vi "AuMT8852B Max Input Power Configuration.vi"(5 "Settings":T1={"Low frequency selection"=enum."Use low frequency", "Medium frequency selection"=enum."Use medium frequency", "High frequency selection"=enum."Use high frequency", "Low TX frequency"=2480.0, "Low RX frequency"=2402.0, "Medium TX frequency"=2402.0, "Medium RX frequency"=2441.0, "High TX frequency"=2402.0, "High RX frequency"=2480.0, "Number of packets"=7408, "Test TX power"=-20.0, "BER limit"=0.1, "FER limit"=100.0, "Packet count"=enum."TX"} {"FER limit" format="%.2f"; "BER limit" format="%.2f"; "Test TX power" format="%.1f"}, 7 "Set/Get (Set)":enum16{"Set", "Get"}(ring), 8 "error in (no error)":errorcluster, 10 "Script (3)":i32=3, 11 "VISA session":refnum<visa-resource-name>) -> (0 "error out":errorcluster, 2 "error code":i32, 3 "VISA session out":refnum<visa-resource-name>, 4 "Settings out":T1={"Low frequency selection"=enum."Use low frequency", "Medium frequency selection"=enum."Use medium frequency", "High frequency selection"=enum."Use high frequency", "Low TX frequency"=0.0, "Low RX frequency"=0.0, "Medium TX frequency"=0.0, "Medium RX frequency"=0.0, "High TX frequency"=0.0, "High RX frequency"=0.0, "Number of packets"=0, "Test TX power"=0.0, "BER limit"=0.0, "FER limit"=0.0, "Packet count"=enum."TX"} {"FER limit" format="%.2f"; "BER limit" format="%.2f"; "Test TX power" format="%.1f"})   [LabVIEW 2017]
doc: "Anritsu MT8852B Bluetooth Tester\n\nConfigures the instrument for the Maximum Input Power Sensitivity test.\n\nINPUTS\nSet/Get - whether the values are being sent to or retrieved from the instrument.\nScript - which of the stored scripts (1-10) will be queried or configured. Scripts 1 and 2 are read-only.\nSettings - parameters of the test to be written.\n\nOUTPUTS\nSettings out - current parameters of the test."
uses:
  <instrlib>/aumt8852B/General/Utilities/MT8850 Test Parameters.ctl
  <instrlib>/aumt8852B/General/Utilities/MT8850 Frequency Units.ctl
panel:
  in  "Case Constant\n(See Context Help)":bool
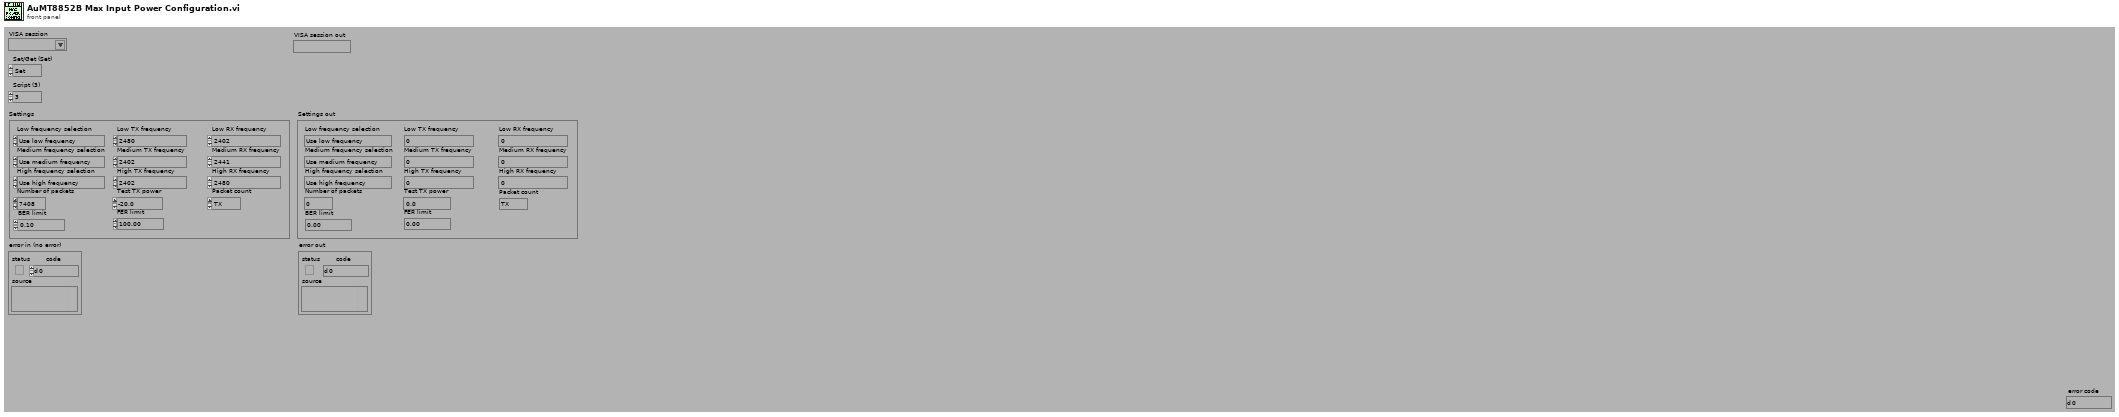
[diagram p1: front panel]
types:
  T1 = cluster{"Low frequency selection":enum16{"Don't use low frequency", "Use low frequency"}, "Medium frequency selection":enum16{"Don't use medium frequency", "Use medium frequency"}, "High frequency selection":enum16{"Don't use high frequency", "Use high frequency"}, "Low TX frequency":dbl, "Low RX frequency":dbl, "Medium TX frequency":dbl, "Medium RX frequency":dbl, "High TX frequency":dbl, "High RX frequency":dbl, "Number of packets":i32, "Test TX power":dbl, "BER limit":dbl, "FER limit":dbl, "Packet count":enum16{"TX", "RX"}}
  T2 = typedef "MT8850 Test Parameters.ctl" = enum16{"Use low frequency", "Use medium frequency", "Use high frequency", "Low TX frequency", "Low RX frquency", "Medium TX frequency", "Medium RX frequency", "High TX frequency", "High RX frequency", "Number of packets", "Average high limit", "Average low limit", "Peak power limit", "Max power step limit", "Min power step limit", "f1 average minimum", "f1 average maximum", "f2 maximum", "f1/f2 average maximum", "Hop selection", "Use DH1 packets", "Use DH3 packets", "Use DH5 packets", "1 slot packet drift limit", "3 slot packet drift limit", "5 slot packet drift limit", "Drift rate limit", "TX power level", "Frequency offset", "Symbol timing", "Modulation index", "BER limit", "FER limit", "Use averaging high limit", "Use averaging low limit", "Use peak power limit", "Packet type", "Test control", "Use max power step limit", "Use min power step limit", "Number of cycles", "Use f1 average maximum", "Use f1 average minimum", "Use f2 maximum", "Use f1/f2 average maximum", "Hop mode", "Maximum negative limit", "Maximum positive limit", "Use maximum negative limit", "Use maximum positive limit", "Use 1 slot packet drift limit", "Use 3 slot packet drift limit", "Use 5 slot packet drift limit", "Use drift rate limit", "Use BER limit", "Use FER limit", "Use dirty parameter table", "Use null packet drift limit", "Null packet drift limit", "Minimum power", "Power delay", "Packet count", "Payload toggle", "Output power level", "2DHX packet type", "3DHX packet type", "Number of blocks", "TX and RX low frequency", "TX and RX medium frequency", "TX and RX high frequency", "TX frequency", "RX frequency", "Threshold bit count", "Total test bit count", "Number of bits", "PDPSK to PGFSK lower limit", "PDPSK to PGFSK upper limit", "Initial frequency error upper limit", "Initial frequency error lower limit", "Frequency error upper limit", "Frequency error lower limit", "Block frequency error upper limit", "Block frequency error lower limit", "2Mbs RMS DEVM limit", "3Mbs RMS DEVM limit", "2Mbs Peak DEVM limit", "3Mbs Peak DEVM limit", "2Mbs 99% packets DEVM limit", "3Mbs 99% packets DEVM limit", "Percentage of no error packets limit", "Threshold error limit", "Total test error limit"}
  T3 = typedef "MT8850 Frequency Units.ctl" = enum16{"Channel", "Hz", "kHz", "MHz", "GHz"}
  T4 = enum16{"Simulate", "Range check", "Cache", "Query instrument status"}
  T5 = enum16{"Output power", "Power control", "Modulation characteristics", "Initial carrier", "Carrier drift", "Single slot sensitivity", "Multiple slot sensitivity", "Maximum input power"}
  T6 = enum16{"Don't use high frequency", "Use high frequency"}
  T7 = enum16{"Don't use medium frequency", "Use medium frequency"}
  T8 = enum16{"Don't use low frequency", "Use low frequency"}
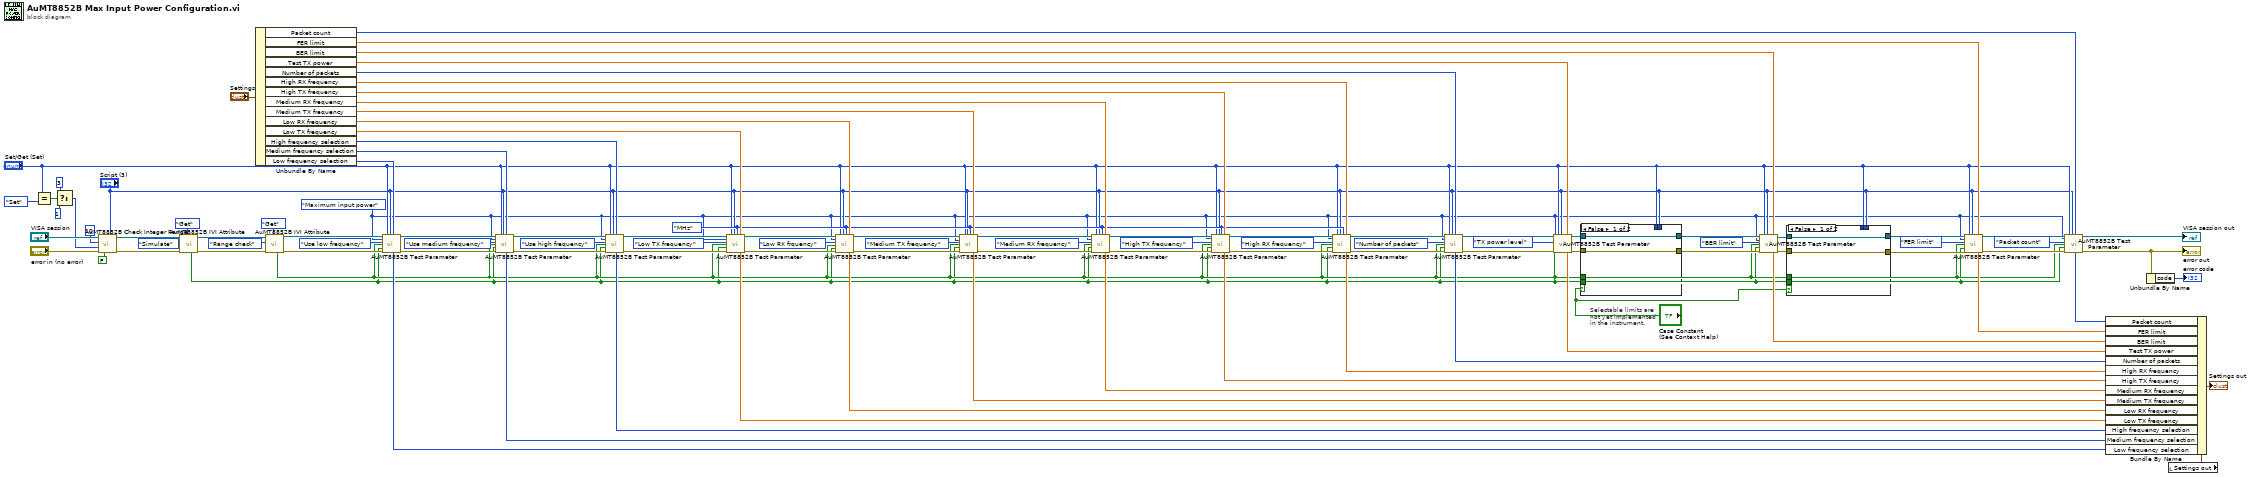
[diagram p0: block diagram]
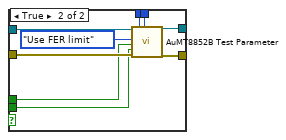
[diagram p2: hidden frame]
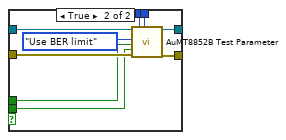
[diagram p3: hidden frame]
diagram:
  w13 = MT8850_Frequency_Units."MHz" ("Frequency units (MHz)")
  w2 = T5."Maximum input power" ("Test (Output Power)")
  # "Selectable limits are\nnot yet implemented\nin the instrument."
  n1 = Equal?(x="Set/Get (Set)", y=enum16{"Set", "Get"}."Set") -> (x = y?=w101:bool)
  n2 = Select(t=3, s=w101, f=1) -> (s? t:f=w97:i32)
  n3 = call <instrlib>:"AuMT8852B Check Integer Range.vi"("Value (0)"="Script (3)", "Check IVI flag first? (T)"=FALSE, "error in (no error)"="error in (no error)", "Lower limit (-1)"=w97, "Upper limit (1)"=10, "VISA session"="VISA session") -> ("error out"=w95:errorcluster, "VISA session out"=w96:refnum<visa-resource-name>)  [unwired: 4 in]
  n4 = call <instrlib>:"AuMT8852B IVI Attribute.vi"("Set/Get (Set)"=enum16{"Set", "Get"}."Get", "error in (no error)"=w95, "Flag (Simulate)"=T4."Simulate", "VISA session"=w96) -> ("error out"=w69:errorcluster, "VISA session out"=w70:refnum<visa-resource-name>, "Value out"=w8:bool)  [unwired: 5 in]
  n5 = Unbundle By Name("Settings") -> ("Packet count"=w1:enum16{"TX", "RX"}, "FER limit"=w37:dbl, "BER limit"=w38:dbl, "Test TX power"=w42:dbl, "Number of packets"=w43:i32, "High RX frequency"=w56:dbl, "High TX frequency"=w57:dbl, "Medium RX frequency"=w44:dbl, "Medium TX frequency"=w58:dbl, "Low RX frequency"=w59:dbl, "Low TX frequency"=w60:dbl, "High frequency selection"=w61:T6, "Medium frequency selection"=w62:T7, "Low frequency selection"=w63:T8)
  n6 = call <instrlib>:"AuMT8852B IVI Attribute.vi"("Set/Get (Set)"=enum16{"Set", "Get"}."Get", "error in (no error)"=w69, "Flag (Simulate)"=T4."Range check", "VISA session"=w70) -> ("error out"=w67:errorcluster, "VISA session out"=w68:refnum<visa-resource-name>, "Value out"=w9:bool)  [unwired: 5 in]
  n7 = call <instrlib>:"AuMT8852B Test Parameter.vi"("VISA session"=w68, "Test (Output power)"=w2, "Parameter (Use low frequency)"=MT8850_Test_Parameters."Use low frequency", "Range check? (F)"=w9, "Simulate? (F)"=w8, "error in (no error)"=w67, "Set/Get (Set)"="Set/Get (Set)", "Script (3)"="Script (3)", "Integer value (0)"=w63) -> ("Integer value out"=w48:i32, "VISA session out"=w20:refnum<visa-resource-name>, "error out"=w19:errorcluster)  [unwired: 7 in, 1 out]
  n8 = call <instrlib>:"AuMT8852B Test Parameter.vi"("VISA session"=w20, "Test (Output power)"=w2, "Parameter (Use low frequency)"=MT8850_Test_Parameters."Use medium frequency", "Range check? (F)"=w9, "Simulate? (F)"=w8, "error in (no error)"=w19, "Set/Get (Set)"="Set/Get (Set)", "Script (3)"="Script (3)", "Integer value (0)"=w62) -> ("Integer value out"=w49:i32, "VISA session out"=w18:refnum<visa-resource-name>, "error out"=w17:errorcluster)  [unwired: 7 in, 1 out]
  n9 = call <instrlib>:"AuMT8852B Test Parameter.vi"("VISA session"=w18, "Test (Output power)"=w2, "Parameter (Use low frequency)"=MT8850_Test_Parameters."Use high frequency", "Range check? (F)"=w9, "Simulate? (F)"=w8, "error in (no error)"=w17, "Set/Get (Set)"="Set/Get (Set)", "Script (3)"="Script (3)", "Integer value (0)"=w61) -> ("Integer value out"=w50:i32, "VISA session out"=w91:refnum<visa-resource-name>, "error out"=w90:errorcluster)  [unwired: 7 in, 1 out]
  n10 = call <instrlib>:"AuMT8852B Test Parameter.vi"("VISA session"=w91, "Test (Output power)"=w2, "Parameter (Use low frequency)"=MT8850_Test_Parameters."Low TX frequency", "Range check? (F)"=w9, "Simulate? (F)"=w8, "error in (no error)"=w90, "Set/Get (Set)"="Set/Get (Set)", "Script (3)"="Script (3)", "Integer value (0)"=w13, "Float value (0)"=w60) -> ("Float value out"=w51:dbl, "VISA session out"=w89:refnum<visa-resource-name>, "error out"=w88:errorcluster)  [unwired: 6 in, 1 out]
  n11 = call <instrlib>:"AuMT8852B Test Parameter.vi"("VISA session"=w89, "Test (Output power)"=w2, "Parameter (Use low frequency)"=MT8850_Test_Parameters."Low RX frquency", "Range check? (F)"=w9, "Simulate? (F)"=w8, "error in (no error)"=w88, "Set/Get (Set)"="Set/Get (Set)", "Script (3)"="Script (3)", "Integer value (0)"=w13, "Float value (0)"=w59) -> ("Float value out"=w52:dbl, "VISA session out"=w87:refnum<visa-resource-name>, "error out"=w86:errorcluster)  [unwired: 6 in, 1 out]
  n12 = call <instrlib>:"AuMT8852B Test Parameter.vi"("VISA session"=w87, "Test (Output power)"=w2, "Parameter (Use low frequency)"=MT8850_Test_Parameters."Medium TX frequency", "Range check? (F)"=w9, "Simulate? (F)"=w8, "error in (no error)"=w86, "Set/Get (Set)"="Set/Get (Set)", "Script (3)"="Script (3)", "Integer value (0)"=w13, "Float value (0)"=w58) -> ("Float value out"=w53:dbl, "VISA session out"=w85:refnum<visa-resource-name>, "error out"=w84:errorcluster)  [unwired: 6 in, 1 out]
  n13 = call <instrlib>:"AuMT8852B Test Parameter.vi"("VISA session"=w85, "Test (Output power)"=w2, "Parameter (Use low frequency)"=MT8850_Test_Parameters."Medium RX frequency", "Range check? (F)"=w9, "Simulate? (F)"=w8, "error in (no error)"=w84, "Set/Get (Set)"="Set/Get (Set)", "Script (3)"="Script (3)", "Integer value (0)"=w13, "Float value (0)"=w44) -> ("Float value out"=w46:dbl, "VISA session out"=w83:refnum<visa-resource-name>, "error out"=w82:errorcluster)  [unwired: 6 in, 1 out]
  n14 = call <instrlib>:"AuMT8852B Test Parameter.vi"("VISA session"=w83, "Test (Output power)"=w2, "Parameter (Use low frequency)"=MT8850_Test_Parameters."High TX frequency", "Range check? (F)"=w9, "Simulate? (F)"=w8, "error in (no error)"=w82, "Set/Get (Set)"="Set/Get (Set)", "Script (3)"="Script (3)", "Integer value (0)"=w13, "Float value (0)"=w57) -> ("Float value out"=w54:dbl, "VISA session out"=w81:refnum<visa-resource-name>, "error out"=w80:errorcluster)  [unwired: 6 in, 1 out]
  n15 = call <instrlib>:"AuMT8852B Test Parameter.vi"("VISA session"=w81, "Test (Output power)"=w2, "Parameter (Use low frequency)"=MT8850_Test_Parameters."High RX frequency", "Range check? (F)"=w9, "Simulate? (F)"=w8, "error in (no error)"=w80, "Set/Get (Set)"="Set/Get (Set)", "Script (3)"="Script (3)", "Integer value (0)"=w13, "Float value (0)"=w56) -> ("Float value out"=w55:dbl, "VISA session out"=w79:refnum<visa-resource-name>, "error out"=w78:errorcluster)  [unwired: 6 in, 1 out]
  n16 = call <instrlib>:"AuMT8852B Test Parameter.vi"("VISA session"=w79, "Test (Output power)"=w2, "Parameter (Use low frequency)"=MT8850_Test_Parameters."Number of packets", "Range check? (F)"=w9, "Simulate? (F)"=w8, "error in (no error)"=w78, "Set/Get (Set)"="Set/Get (Set)", "Script (3)"="Script (3)", "Integer value (0)"=w43) -> ("Integer value out"=w45:i32, "VISA session out"=w33:refnum<visa-resource-name>, "error out"=w32:errorcluster)  [unwired: 7 in, 1 out]
  n17 = call <instrlib>:"AuMT8852B Test Parameter.vi"("VISA session"=w33, "Test (Output power)"=w2, "Parameter (Use low frequency)"=MT8850_Test_Parameters."TX power level", "Range check? (F)"=w9, "Simulate? (F)"=w8, "error in (no error)"=w32, "Set/Get (Set)"="Set/Get (Set)", "Script (3)"="Script (3)", "Float value (0)"=w42) -> ("Float value out"=w36:dbl, "VISA session out"=w26:refnum<visa-resource-name>, "error out"=w23:errorcluster)  [unwired: 7 in, 1 out]
  n18 = case shown="False" "Case Constant\n(See Context Help)" {
    tunnel: w26 -> [w106 w114]
    tunnel: [w106 w113] -> w25
    tunnel: [w105 w112] -> w24
    tunnel: w23 -> [w105 w111]
    tunnel: w9 -> [_ w110]
    tunnel: w8 -> [_ w109]
    tunnel: "Set/Get (Set)" -> [_ w108]
    tunnel: "Script (3)" -> [_ w107]
    frame False {
    }
    frame True {
      n19 = call <instrlib>:"AuMT8852B Test Parameter.vi"("VISA session"=w114, "Parameter (Use low frequency)"=MT8850_Test_Parameters."Use BER limit", "Range check? (F)"=w110, "Simulate? (F)"=w109, "error in (no error)"=w111, "Set/Get (Set)"=w108, "Script (3)"=w107) -> ("VISA session out"=w113:refnum<visa-resource-name>, "error out"=w112:errorcluster)  [unwired: 9 in, 2 out]
    }
  }
  n20 = call <instrlib>:"AuMT8852B Test Parameter.vi"("VISA session"=w25, "Test (Output power)"=w2, "Parameter (Use low frequency)"=MT8850_Test_Parameters."BER limit", "Range check? (F)"=w9, "Simulate? (F)"=w8, "error in (no error)"=w24, "Set/Get (Set)"="Set/Get (Set)", "Script (3)"="Script (3)", "Float value (0)"=w38) -> ("Float value out"=w35:dbl, "VISA session out"=w30:refnum<visa-resource-name>, "error out"=w29:errorcluster)  [unwired: 7 in, 1 out]
  n21 = case shown="False" "Case Constant\n(See Context Help)" {
    tunnel: w30 -> [w116 w125]
    tunnel: w29 -> [w117 w124]
    tunnel: [w116 w123] -> w28
    tunnel: [w117 w122] -> w27
    tunnel: w9 -> [_ w121]
    tunnel: w8 -> [_ w120]
    tunnel: "Set/Get (Set)" -> [_ w119]
    tunnel: "Script (3)" -> [_ w118]
    frame False {
    }
    frame True {
      n22 = call <instrlib>:"AuMT8852B Test Parameter.vi"("VISA session"=w125, "Parameter (Use low frequency)"=MT8850_Test_Parameters."Use FER limit", "Range check? (F)"=w121, "Simulate? (F)"=w120, "error in (no error)"=w124, "Set/Get (Set)"=w119, "Script (3)"=w118) -> ("VISA session out"=w123:refnum<visa-resource-name>, "error out"=w122:errorcluster)  [unwired: 9 in, 2 out]
    }
  }
  n23 = call <instrlib>:"AuMT8852B Test Parameter.vi"("VISA session"=w28, "Test (Output power)"=w2, "Parameter (Use low frequency)"=MT8850_Test_Parameters."FER limit", "Range check? (F)"=w9, "Simulate? (F)"=w8, "error in (no error)"=w27, "Set/Get (Set)"="Set/Get (Set)", "Script (3)"="Script (3)", "Float value (0)"=w37) -> ("Float value out"=w34:dbl, "VISA session out"=w12:refnum<visa-resource-name>, "error out"=w11:errorcluster)  [unwired: 7 in, 1 out]
  n24 = call <instrlib>:"AuMT8852B Test Parameter.vi"("VISA session"=w12, "Test (Output power)"=w2, "Parameter (Use low frequency)"=MT8850_Test_Parameters."Packet count", "Range check? (F)"=w9, "Simulate? (F)"=w8, "error in (no error)"=w11, "Set/Get (Set)"="Set/Get (Set)", "Script (3)"="Script (3)", "Integer value (0)"=w1) -> ("Integer value out"=w5:i32, "VISA session out"=→"VISA session out":refnum<visa-resource-name>, "error out"=w7:errorcluster)  [unwired: 7 in, 1 out]
  "error out" <- w7
  n25 = Unbundle By Name(w7) -> ("code"=→"error code":i32)
  n26 = local read "Settings out"() -> (w47:T1)
  n27 = Bundle By Name(cluster=w47, "Packet count"=w5, "FER limit"=w34, "BER limit"=w35, "Test TX power"=w36, "Number of packets"=w45, "High RX frequency"=w55, "High TX frequency"=w54, "Medium RX frequency"=w46, "Medium TX frequency"=w53, "Low RX frequency"=w52, "Low TX frequency"=w51, "High frequency selection"=w50, "Medium frequency selection"=w49, "Low frequency selection"=w48) -> (→"Settings out":T1)
